vi "Get associated LabVIEW error.vi"(11 "IRequestResult in":refnum<class "IRequestResult.lvclass">) -> (2 "LabVIEW Equivalent Error":errorcluster, 3 "IRequestResult out":refnum<class "IRequestResult.lvclass">)   [LabVIEW 2020, in "wamplv.lvlib" / "IRequestResult.lvclass"]
uses:
  IRequestResult.lvclass
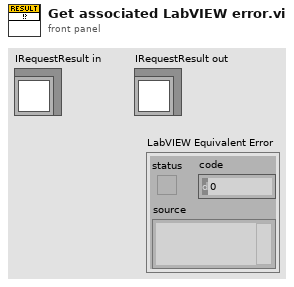
[diagram p1: front panel]
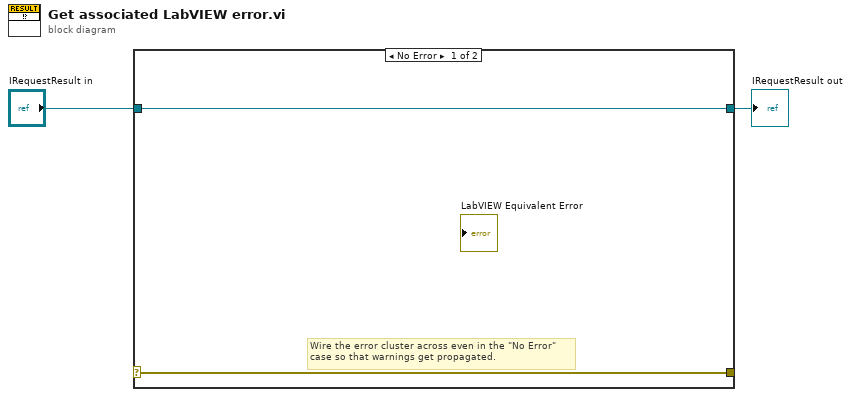
[diagram p0: block diagram]
diagram:
  n1 = case shown="No Error" {
    selector: _ -> [w3 w6]
    tunnel: [w3 w6] -> _
    tunnel: [w4 w5] -> w1
    tunnel: "IRequestResult in" -> [w4 w5]
    frame No Error {
      # "Wire the error cluster across even in the \"No Error\"\ncase so that warnings get propagated."
    }
    frame Error {
    }
  }
  "IRequestResult out" <- w1
